vi "Initial File Name & Calling VI.vi"() -> (0 "error out":errorcluster, 1 "Calling VI Name":string, 2 "Backup File Name":string, 3 "Default File Name":string)   [LabVIEW 2021, in "Notebook.lvlib"]
uses:
  Notebook.lvlib
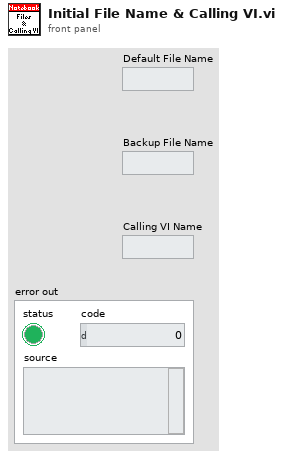
[diagram p1: front panel]
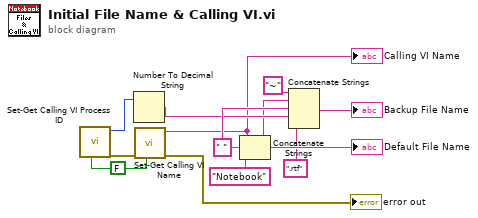
[diagram p0: block diagram]
diagram:
  w1 = FALSE ("Set/Get (F)")
  w12 = " " ("string")
  n1 = call "Set-Get Calling VI Process ID.vi"("Set/Get (F)"=w1) -> ("Error Out"=w9:errorcluster, "ProcessID"=w10:u32)  [unwired: 9 in]
  n2 = Number To Decimal String(number=w10) -> (decimal integer string=w11:string)  [unwired: 1 in]
  n3 = call "Set-Get Calling VI Name.vi"("Set/Get (F)"=w1, "Error In"=w9) -> ("Error Out"=→"error out":errorcluster, "Calling VI Name"=w8:string)  [unwired: 8 in]
  "Calling VI Name" <- w8
  n4 = Concatenate Strings(w8, w12, "Notebook" ("string")) -> (w7:string)
  "Default File Name" <- w7
  n5 = Concatenate Strings("~" ("string"), w7, w12, w11, ".rtf" ("format string")) -> (→"Backup File Name":string)
